vi "SVPO Power Spectrum (N Ch DBL WDT).vi"(0 "scaled signals [EU]":waveform(dbl)[](array[waveform]), 2 "window":T8=1 items=["None"=0, "Hanning"=1, "Hamming"=2, "Blackman-Harris"=3, "Exact Blackman"=4, "Blackman"=5, "Flat Top"=6, "4 Term B-Harris "=7, "7 Term B-Harris"=8, "Low Sidelobe"=9, "Force"=64, "Exponential"=65, "Blackman Nuttall"=11, "Triangle"=30, "Bartlett-Hanning"=31, "Bohman"=32, "Parzen"=33, "Welch"=34, "Kaiser"=60, "Dolph-Chebyshev"=61, "Gaussian"=62], 9 "restart averaging? (F)":bool) -> (13 "averages completed":dbl, 14 "power spectra [EU^2 rms]":T7(array[cluster]) {"magnitude" format="%.2p"; "df [Hz]" format="%.2p"; "f0 [Hz]" format="%.2p"}, 18 "spectrum info":T1={"channel name"="", "description"="", "x-axis units"=0, "spectral info"={"spectrum type"=enum."Power [Magnitude^2]", "linear/dB"=enum."linear", "window"=0, "window size"=0, "FFT size"=0}, "engineering units"=0, "custom label"="", "dB reference [EU]"=0.0, "peak units"=enum."rms", "weighting filter"=0, "spectral density?"=FALSE, "unit label"="", "spectrum skewed?"=FALSE, "complimentary spectrum units"=enum."none"} {"x-axis units" items=["Time (s)"=0, "Frequency-CB (Hz)"=1, "Frequency-CPB (Hz)"=1248, "Frequency-Arbitrary (Hz)"=2357, "Quefrency (s)"=2, "Revolutions (rev)"=3, "Order"=4, "Speed (RPM)"=11, "Speed (rad/s)"=21, "Index"=65535]; "weighting filter" items=["Linear", "A-weighting", "B-weighting", "C-weighting", "ITU-R 468-4", "Dolby", "CCITT", "C-message", "Wb", "Wc", "Wd", "We", "Wf", "Wh", "Wj", "Wk", "Wm", "AES17 20 kHz lowpass", "AES17 40 kHz lowpass", "AES17 20 kHz highpass", "AES17 40 kHz highpass"]; "dB reference [EU]" format="%.2f"; "engineering units" items=["custom..."=0, "V"=1, "A"=21, "C"=30, "pC"=31, "s"=32, "-"=29, "Pa"=2, "N"=20, "g"=3, "m/s^2"=4, "m/s"=5, "m"=6, "mm/s"=12, "mm"=13, "micron/s"=14, "micron"=15, "in/s^2"=7, "in/s"=8, "in"=9, "mil/s"=10, "mil"=11, "rad/s^2"=16, "rad/s"=17, "rad"=18, "deg/s^2"=26, "deg/s"=27, "deg"=28, "RPM"=22, "cycle/s^2"=23, "Hz"=24, "cycle"=25, "strain"=19]; "spectral info"."window" items=["None "=0, "Hanning"=1, "Hamming"=2, "Blackman-Harris"=3, "Exact Blackman"=4, "Blackman"=5, "Flat Top"=6, "4 Term B-Harris "=7, "7 Term B-Harris"=8, "Low Sidelobe"=9, "Force - Exponential"=10, "Gaussian"=62]})   [LabVIEW 2017]
doc: "Computes the linear RMS-averaged power spectrum of <B>scaled signal [EU]</B> in a linear scale. Use the power spectrum to quantify signal components as a function of frequency. Use this VI on embedded targets that have limited computational resources. Wire data to the <B>scaled signal [EU]</B> input to determine the polymorphic instance to use or manually select the instance."
uses:
  <vilib>/addons/_NISVFA/_Shared subVIs/Controls/svc_Window.ctl
  <vilib>/addons/_NISVFA/_Shared subVIs/Controls/svc_Spectrum Info.ctl
  <vilib>/addons/_NISVFA/_Shared subVIs/Controls/svc_X-Axis Units.ctl
  <vilib>/addons/_NISVFA/_Shared subVIs/Controls/svc_Spectrum Type.ctl
  <vilib>/addons/_NISVFA/_Shared subVIs/Controls/svc_Engineering Units Text Ring.ctl
  <vilib>/addons/_NISVFA/_Shared subVIs/Controls/svc_Weighting Filter Text Ring.ctl
  <vilib>/addons/_NISVFA/_Shared subVIs/Controls/svc_Complimentary Spectrum Units.ctl
  <vilib>/Analysis/2dsp.llb/Power Spectrum (DBL).vi
  <vilib>/Analysis/4window.llb/Force Window.vi
  <vilib>/Analysis/4window.llb/Force Window (DBL).vi
  <vilib>/Analysis/4window.llb/Exponential Window.vi
  <vilib>/Analysis/4window.llb/Exponential Window (DBL).vi
  <vilib>/Utility/error.llb/Error Cluster From Error Code.vi
  <vilib>/Analysis/0measdsp.llb/Scaled Time Domain Window.vi
  <vilib>/Analysis/0measdsp.llb/Scaled Time Domain Window (DBL).vi
  <vilib>/addons/_NISVFA/_Spectrum Processing/subVIs/svfa_Spectrum Info Window to windowTd Type Def.vi
  <vilib>/Analysis/NI_AALPro.lvlib
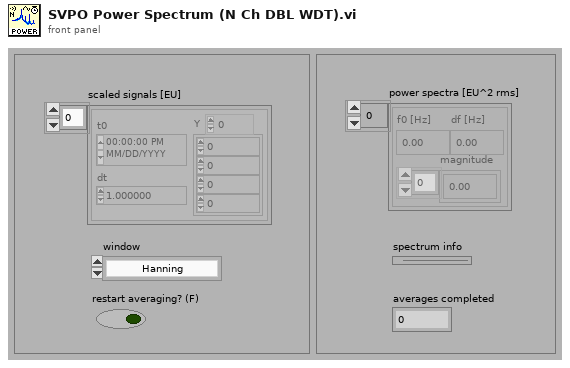
[diagram p1: front panel]
types:
  T1 = typedef "svc_Spectrum Info.ctl" = cluster{"channel name":string, "description":string, "x-axis units":T2, "spectral info":cluster{"spectrum type":T3, "linear/dB":enum16{"linear", "dB"}, "window":u16, "window size":i32, "FFT size":i32}, "engineering units":T4, "custom label":string, "dB reference [EU]":dbl, "peak units":enum16{"rms", "peak", "peak-peak"}, "weighting filter":T5, "spectral density?":bool, "unit label":string, "spectrum skewed?":bool, "complimentary spectrum units":T6}
  T2 = typedef "svc_X-Axis Units.ctl" = u16
  T3 = typedef "svc_Spectrum Type.ctl" = enum16{"FFT Spectrum [complex]", "Amplitude [Magnitude]", "Power [Magnitude^2]", "Cross Spectrum [complex]", "Frequency Response [Complex]"}
  T4 = typedef "svc_Engineering Units Text Ring.ctl" = u16
  T5 = typedef "svc_Weighting Filter Text Ring.ctl" = u16
  T6 = typedef "svc_Complimentary Spectrum Units.ctl" = enum16{"none", "radians", "degrees", "cycles", "imaginary"}
  T7 = cluster{"f0 [Hz]":dbl, "df [Hz]":dbl, "magnitude":dbl[]}[]
  T8 = typedef "svc_Window.ctl" = u32
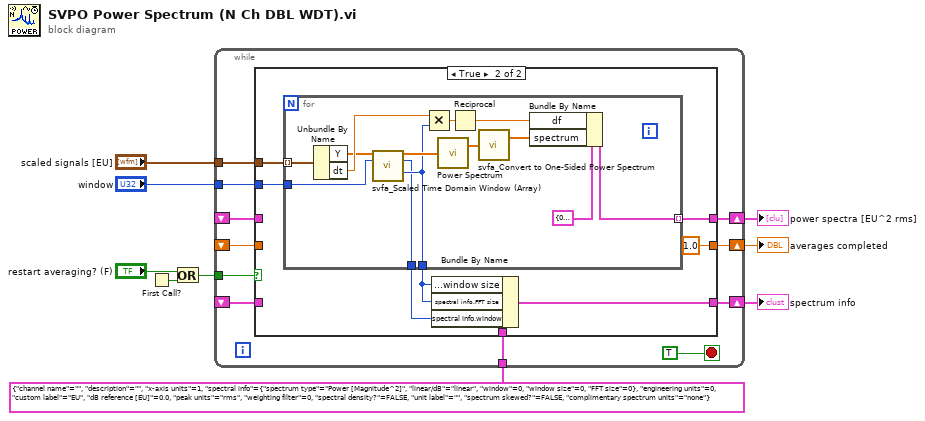
[diagram p0: block diagram]
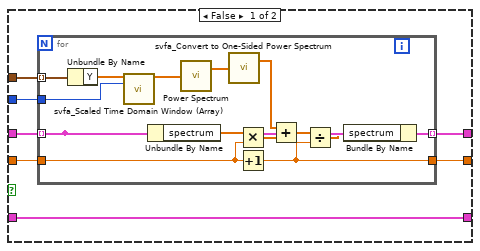
[diagram p2: hidden frame]
diagram:
  n1 = First Call?() -> (First Call?: T/F=w5:bool)
  n2 = Or(x="restart averaging? (F)", y=w5) -> (x .or. y?=w4:bool)
  n3 = while {
    tunnel: "window" -> [w16]
    shift-left: _ -> [w17]
    shift-right: [w18] -> w1
    tunnel: w4 -> [w14]
    tunnel: "scaled signals [EU]" -> [w19]
    tunnel: T1 {"channel name"="", "description"="", "x-axis units"=1, "spectral info"={"spectrum type"=enum."Power [Magnitude^2]", "linear/dB"=enum."linear", "window"=0, "window size"=0, "FFT size"=0}, "engineering units"=0, "custom label"="EU", "dB reference [EU]"=0.0, "peak units"=enum."rms", "weighting filter"=0, "spectral density?"=FALSE, "unit label"="", "spectrum skewed?"=FALSE, "complimentary spectrum units"=enum."none"} ("spectrum info in") -> [w13]
    shift-right: [w12] -> w2
    shift-left: _ -> [w11]
    shift-right: [w15] -> w7
    shift-left: _ -> [w10]
    stop <- TRUE stop-if-true
    n4 = case shown="True" w14 {
      tunnel: w19 -> [w26 w49]
      tunnel: [w24 1.0 ("f0")] -> w18
      tunnel: w17 -> [w27 _]
      tunnel: w16 -> [w25 w43]
      tunnel: [w23 w48] -> w15
      tunnel: w13 -> [_ w47]
      tunnel: [w22 w45] -> w12
      tunnel: w11 -> [w22 _]
      tunnel: w10 -> [w21 _]
      frame False {
        n5 = for {
          tunnel: w27 -> [w32]
          tunnel: w26 -> [w41] mode=indexing
          tunnel: w25 -> [w37]
          tunnel: [w28] -> w24
          tunnel: [w29] -> w23 mode=indexing
          tunnel: w21 -> [w31] mode=indexing
          n6 = Unbundle By Name ("Get Waveform Components")(w41) -> ("Y"=w39:dbl[])
          n7 = call <vilib>:"svfa_Scaled Time Domain Window (Array).vi"("input signal"=w39, "window"=w37) -> ("windowed signal"=w38:dbl[])  [unwired: 8 in, 5 out]
          n8 = Unbundle By Name(w31) -> ("spectrum"=w33:dbl[])
          n9 = call-poly <vilib>:"Power Spectrum.vi"("X"=w38) -> ("Power Spectrum"=w40:dbl[])  [unwired: 1 out]
          n10 = call <vilib>:"svfa_Convert to One-Sided Power Spectrum.vi"("two-sided power spectrum"=w40) -> ("one-sided power spectrum"=w34:dbl[])  [unwired: 1 out]
          n11 = Multiply(x=w33, y=w32) -> (x*y=w36:dbl[])
          n12 = Increment(x=w32) -> (x+1=w28:dbl)
          n13 = Add(x=w34, y=w36) -> (x+y=w35:dbl[])
          n14 = Divide(x=w35, y=w28) -> (x/y=w30:dbl[])
          n15 = Bundle By Name(cluster=w31, "spectrum"=w30) -> (w29:cluster{"f0":dbl, "df":dbl, "spectrum":dbl[]})
        }
      }
      frame True {
        n16 = for {
          tunnel: w49 -> [w59] mode=indexing
          tunnel: [w58] -> w48 mode=indexing
          tunnel: w43 -> [w56]
          tunnel: [w53] -> w46
          tunnel: [w52] -> w42
          n17 = Unbundle By Name ("Get Waveform Components")(w59) -> ("Y"=w57:dbl[], "dt"=w61:dbl)
          n18 = call <vilib>:"svfa_Scaled Time Domain Window (Array).vi"("input signal"=w57, "window"=w56) -> ("windowed signal"=w55:dbl[], "dup window"=w52:T8, "FFT length"=w53:i32)  [unwired: 8 in, 3 out]
          n19 = Multiply(x=w61, y=w53) -> (x*y=w62:dbl)
          n20 = call-poly <vilib>:"Power Spectrum.vi"("X"=w55) -> ("Power Spectrum"=w60:dbl[])  [unwired: 1 out]
          n21 = Reciprocal(x=w62) -> (1/x=w51:dbl)
          n22 = call <vilib>:"svfa_Convert to One-Sided Power Spectrum.vi"("two-sided power spectrum"=w60) -> ("one-sided power spectrum"=w54:dbl[])  [unwired: 1 out]
          n23 = Bundle By Name(cluster=cluster{"f0":dbl, "df":dbl, "spectrum":dbl[]} {"f0"=0.0, "df"=0.0, "spectrum"=[]}, "df"=w51, "spectrum"=w54) -> (w58:cluster{"f0":dbl, "df":dbl, "spectrum":dbl[]})
        }
        n24 = Bundle By Name(cluster=w47, "spectral info.window size"=w46, "spectral info.FFT size"=w46, "spectral info.window"=w42) -> (w45:T1)
      }
    }
  }
  "power spectra [EU^2 rms]" <- w7
  "spectrum info" <- w2
  "averages completed" <- w1
